vi "AutoNetwork.vi"   [LabVIEW 2020]
uses:
  AutoGlobals.vi
  <vilib>/Rock Robotics/Network Tables/NT Write Number.vi
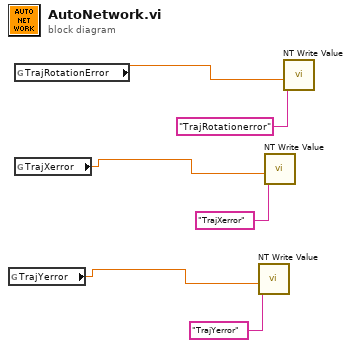
[diagram p0: block diagram]
diagram:
  n1 = global read "AutoGlobals.vi" "TrajYerror"() -> (w3:dbl)
  n2 = global read "AutoGlobals.vi" "TrajRotationError"() -> (w1:dbl)
  n3 = global read "AutoGlobals.vi" "TrajXerror"() -> (w5:dbl)
  n4 = call-poly <vilib>:"NT Write Value.vi"("Numeric"=w3, "Name"="TrajYerror") -> ()  [unwired: 9 in, 1 out]
  n5 = call-poly <vilib>:"NT Write Value.vi"("Numeric"=w5, "Name"="TrajXerror") -> ()  [unwired: 9 in, 1 out]
  n6 = call-poly <vilib>:"NT Write Value.vi"("Numeric"=w1, "Name"="TrajRotationerror") -> ()  [unwired: 9 in, 1 out]
